vi "BuildPlotColorsBands.vi"(5 "Labels":string[](array[string]), 6 "View Type":u16(ring) items=["As measured", "Normalize", "Separate", "Cplx Average", "Real Average", "Standard Deviation"], 7 "Colors":u32[](array[numeric]), 8 "error in (no error)":errorcluster, 9 "Bands":u16, 11 "WaveformGraph in":refnum<vi>) -> (3 "WaveformGraph out":refnum<vi>)   [LabVIEW 2022 SP3]
uses:
  Mic/Mic_Global.vi
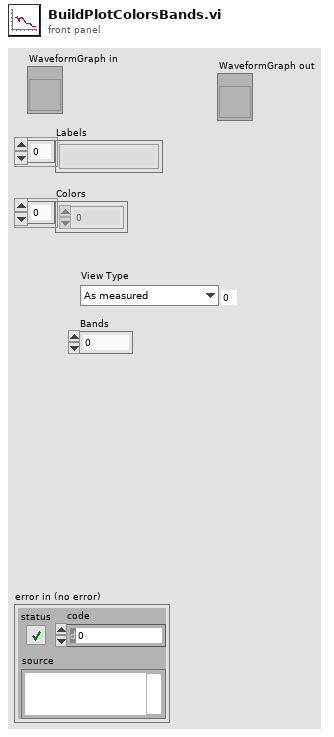
[diagram p1: front panel]
types:
  T1 = cluster{"Alerts":bool, "Log X Axis":bool, "dB scale":bool, "Averaging":bool, "Fade":dbl, "Centroids?":bool}
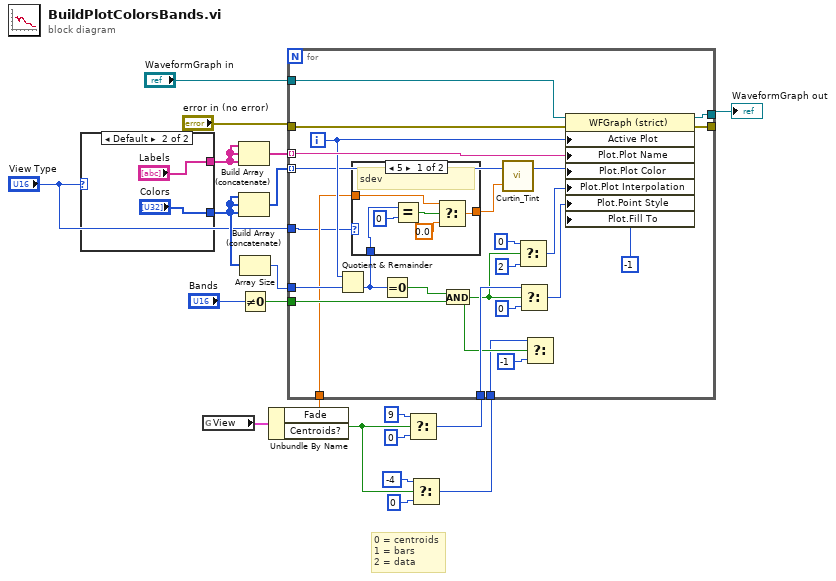
[diagram p0: block diagram]
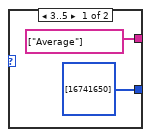
[diagram p2: hidden frame]
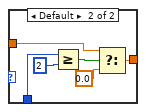
[diagram p3: hidden frame]
diagram:
  # "0 = centroids\n1 = bars\n2 = data"
  n1 = case shown="Default" "View Type" {
    tunnel: [string[] ["Average"] ("Labels") "Labels"] -> w12
    tunnel: [u32[] [16741650] ("Colors") "Colors"] -> w11
    frame 3..5 {
    }
    frame Default {
    }
  }
  n2 = global read "Mic_Global.vi" "View"() -> (w10:T1)
  n3 = Build Array (concatenate)(w12, w12, w12) -> (w17:string[])
  n4 = Build Array (concatenate)(w11, w11, w11) -> (w14:u32[])
  n5 = Array Size(array=w11) -> (size(s)=w15:i32)
  n6 = Not Equal To 0?(x="Bands") -> (x != 0?=w20:bool)
  n7 = Unbundle By Name(w10) -> ("Fade"=w6:dbl, "Centroids?"=w3:bool)
  n8 = Select(t=9 ("y"), s=w3, f=0 ("y")) -> (s? t:f=w7:i32)
  n9 = Select(t=-4 ("y"), s=w3, f=0 ("y")) -> (s? t:f=w2:i32)
  n10 = for {
    tunnel: w14 -> [w32] mode=indexing
    tunnel: "WaveformGraph in" -> [w49]
    tunnel: w15 -> [w41]
    tunnel: "error in (no error)" -> [w46]
    tunnel: [w45] -> _
    tunnel: w17 -> [w44] mode=indexing
    tunnel: [w43] -> w18
    tunnel: w20 -> [w40]
    tunnel: w7 -> [w31]
    tunnel: w6 -> [w30]
    tunnel: w2 -> [w27]
    tunnel: "View Type" -> [w25]
    i -> [w42]
    n11 = Quotient & Remainder(x=w42, y=w41) -> (floor(x/y)=w39:i32)  [unwired: 1 out]
    n12 = case shown="5" w25 {
      tunnel: [w51 w61] -> w48
      tunnel: w39 -> [w50 w57]
      tunnel: w30 -> [w52 w56]
      frame 5 {
        # "sdev"
        n13 = Equal?(x=w50, y=0) -> (x = y?=w54:bool)
        n14 = Select(t=w52, s=w54, f=0.0 ("t")) -> (s? t:f=w51:dbl)
      }
      frame Default {
        n15 = Greater Or Equal?(x=w57, y=2) -> (x >= y?=w59:bool)
        n16 = Select(t=w56, s=w59, f=0.0 ("t")) -> (s? t:f=w61:dbl)
      }
    }
    n17 = Equal To 0?(x=w39) -> (x = 0?=w38:bool)
    n18 = And(x=w38, y=w40) -> (x .and. y?=w28:bool)
    n19 = call "Curtin_Tint.vi"("Tint Factor"=w48, "Plot.Plot Color"=w32) -> ("Plot.Plot Color 2"=w47:u32)  [unwired: 1 in]
    n20 = Select(t=0 ("y"), s=w28, f=2 ("y")) -> (s? t:f=w33:i32)
    n21 = Select(t=w31, s=w28, f=0 ("y")) -> (s? t:f=w36:i32)
    n22 = Select(t=w27, s=w28, f=-1 ("y")) -> ()  [unwired: 1 out]
    n23 = property on="Property Node" class="WFGraph (strict)"(reference=w49, error in=w46, "Active Plot"=w42, "Plot.Plot Name"=w44, "Plot.Plot Color"=w47, "Plot.Plot Interpolation"=w33, "Plot.Point Style"=w36, "Plot.Fill To"=i16 -1) -> (reference out=w43:refnum<vi>, error out=w45:errorcluster)
  }
  "WaveformGraph out" <- w18
